vi "SSL Detection Points Referee.vi"(8 "error in":errorcluster, 9 "Array":u8[](array[numeric]) format="%02x") -> (0 "error out":errorcluster, 1 "Length-delimited":u8[](array[numeric]) format="%02x", 3 "Point":cluster{"x":sgl, "y":sgl})   [LabVIEW 2016]
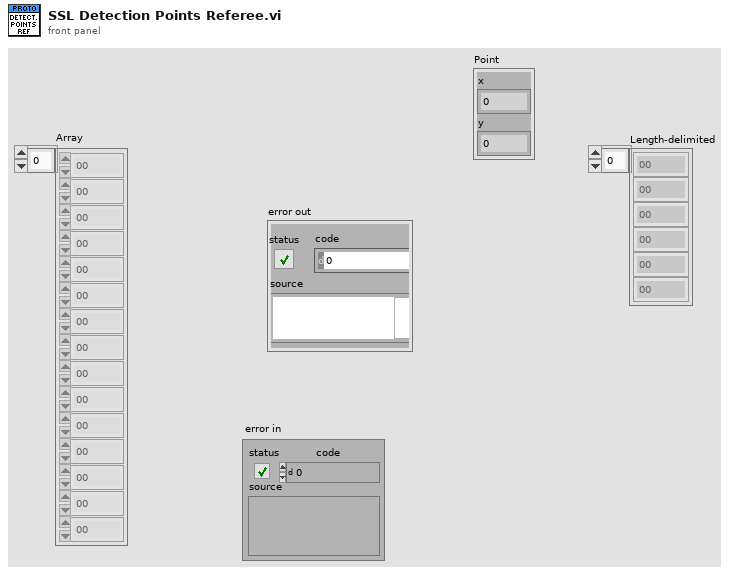
[diagram p1: front panel]
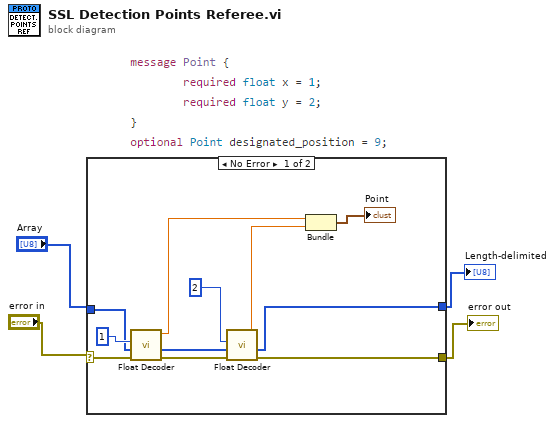
[diagram p0: block diagram]
diagram:
  n1 = case shown="No Error" "error in" {
    selector: "error in" -> [w15 w17]
    tunnel: [w13 w17] -> w3
    tunnel: [w8 w16] -> w2
    tunnel: "Array" -> [w10 w16]
    frame No Error {
      n2 = call "Float Decoder.vi"("error in (no error)"=w15, "Array"=w10, "Key"=1) -> ("error out"=w14:errorcluster, "array w/ subset deleted"=w9:u8[], "Float"=w7:sgl)  [unwired: 5 in, 1 out]
      n3 = call "Float Decoder.vi"("error in (no error)"=w14, "Array"=w9, "Key"=2) -> ("error out"=w13:errorcluster, "array w/ subset deleted"=w8:u8[], "Float"=w6:sgl)  [unwired: 5 in, 1 out]
      n4 = Bundle("Float"=w7, "Float"=w6) -> (→"Point":cluster{"Float":sgl, "Float":sgl})  [unwired: 1 in]
    }
    frame Error {
    }
  }
  "error out" <- w3
  "Length-delimited" <- w2
